vi "Protocol Component Matches Special Scheme.vi"(11 "Component":T1) -> (3 "Special Scheme":bool)   [LabVIEW 2020, in "Stream.lvlib" / "URLPattern.lvclass"]
uses:
  URLPattern.lvclass
  Component.ctl
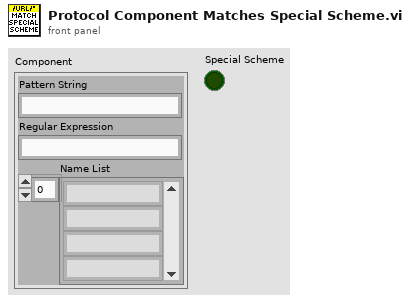
[diagram p1: front panel]
types:
  T1 = typedef "Stream.lvlib/URLPattern.lvclass/Component.ctl" = cluster{"Pattern String":string, "Regular Expression":string, "Name List":string[]}
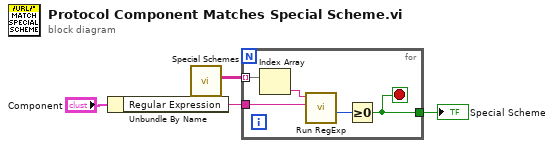
[diagram p0: block diagram]
diagram:
  n1 = Unbundle By Name("Component") -> ("Regular Expression"=w2:string)
  n2 = call "Special Schemes.vi"() -> ("Special Schemes"=w4:string[][])  [unwired: 11 in]
  n3 = for {
    tunnel: w4 -> [w9] mode=indexing
    tunnel: w2 -> [w8]
    tunnel: [w5] -> w1
    stop <- w5 stop-if-true
    n4 = Index Array(array=w9) -> (element=w7:string)  [unwired: 1 in]
    n5 = call "Run RegExp.vi"("regular expression"=w8, "string"=w7) -> ("offset past match"=w6:i32)  [unwired: 5 in, 4 out]
    n6 = Greater Or Equal To 0?(x=w6) -> (x >= 0?=w5:bool)
  }
  "Special Scheme" <- w1
